vi "Subscriber-3.vi"() -> ()   [LabVIEW 2015]
uses:
  <vilib>/Distrio/LabbitMQ/Channel/exchange_type_enum.ctl
  <vilib>/Distrio/LabbitMQ/Connection/Connection.lvclass
  <vilib>/Distrio/LabbitMQ/Connection/connection_parameters_cluster.ctl
  <vilib>/Distrio/LabbitMQ/Queue/Queue.lvclass
  <vilib>/Distrio/LabbitMQ/Channel/Channel.lvclass
panel:
  in  "buttonStop":bool
  out "Received Message":string
  in  "Subscribe":bool
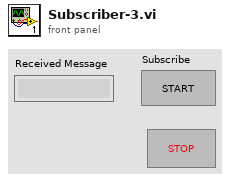
[diagram p1: front panel]
types:
  T1 = typedef "Connection.lvclass/connection_parameters_cluster.ctl" = cluster{"host name":string, "port":i32, "user name":string, "password":string, "virtual host":string}
  T2 = typedef "Channel.lvclass/exchange_type_enum.ctl" = enum16{"direct", "topic", "fanout", "headers"}
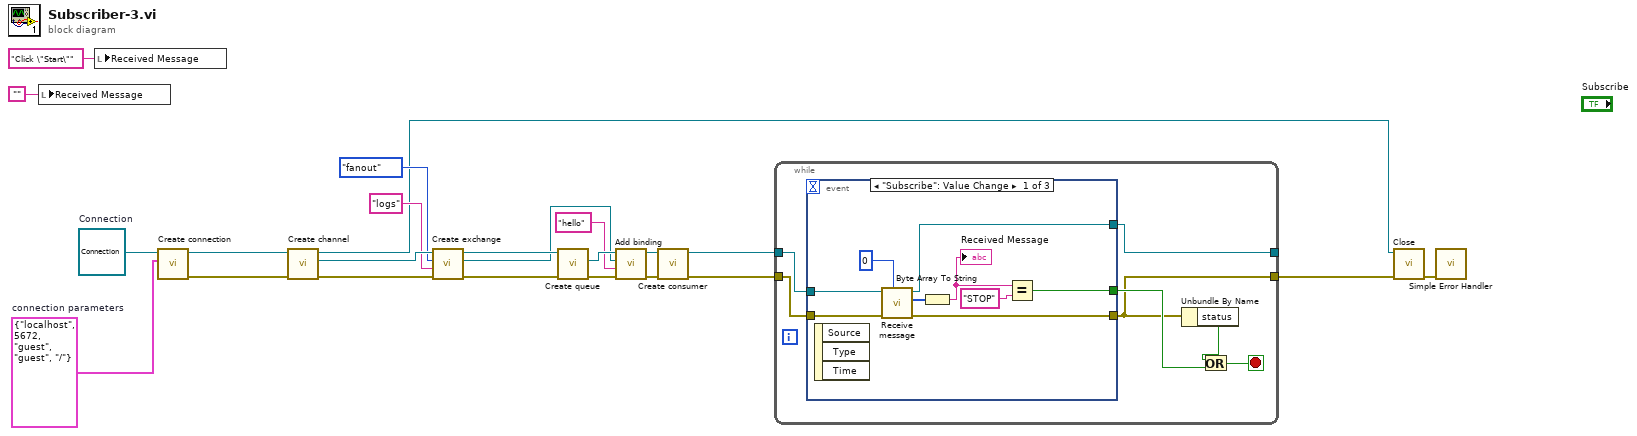
[diagram p0: block diagram]
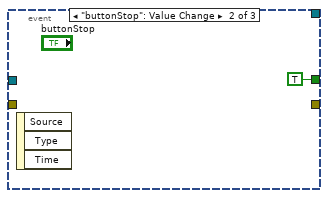
[diagram p2: hidden frame]
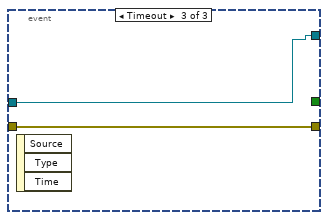
[diagram p3: hidden frame]
diagram:
  w8 = T1 {"host name"="localhost", "port"=5672, "user name"="guest", "password"="guest", "virtual host"="/"}  # connection parameters
  w9 = refnum<class "Connection.lvclass"> refnum  # Connection
  n1 = local write "Received Message"("") -> ()
  n2 = local write "Received Message"("Click \"Start\"") -> ()
  n3 = call <vilib>:"Create connection.vi"("connection parameters"=w8, "Connection in"=w9) -> ("error out"=w22:errorcluster, "Connection out"=w23:refnum<class "Connection.lvclass">)  [unwired: 8 in]
  n4 = call <vilib>:"Create channel.vi"("error in (no error)"=w22, "Connection in"=w23) -> ("error out"=w21:errorcluster, "channel"=w20:refnum<class "Channel.lvclass">, "Connection out"=w7:refnum<class "Connection.lvclass">)  [unwired: 7 in]
  n5 = call <vilib>:"Create exchange.vi"("error in (no error)"=w21, "exchange name"="logs", "exchange type"=exchange_type_enum."fanout" ("binding"), "Channel in"=w20) -> ("error out"=w19:errorcluster, "Exchange.lvclass"=w15:refnum<class "Exchange.lvclass">, "Channel out"=w18:refnum<class "Channel.lvclass">)  [unwired: 5 in]
  n6 = call <vilib>:"Create queue.vi"("error in (no error)"=w19, "Channel in"=w18) -> ("error out"=w17:errorcluster, "Queue.lvclass"=w16:refnum<class "Queue.lvclass">)  [unwired: 7 in, 1 out]
  n7 = call <vilib>:"Add binding.vi"("error in (no error)"=w17, "binding key"="hello" ("routing key"), "Exchange.lvclass"=w15, "Consumer in"=w16) -> ("error out"=w13:errorcluster, "Consumer out"=w12:refnum<class "Queue.lvclass">)  [unwired: 6 in]
  n8 = call <vilib>:"Create consumer.vi"("error in (no error)"=w13, "Queue in"=w12) -> ("error out"=w4:errorcluster, "Queue out"=w5:refnum<class "Queue.lvclass">)  [unwired: 8 in]
  n9 = while {
    tunnel: w5 -> [w30]
    tunnel: w4 -> [w29]
    tunnel: [w25] -> w3
    tunnel: [w28] -> _
    stop <- w26 stop-if-true
    n10 = event shown="[0] \"Subscribe\": Value Change" {
      selector: _ -> [_ _ _]
      dyn-events: _ -> [_ _ _]
      timeout: _ -> [_ _ _]
      tunnel: w30 -> [w38 _ w42]
      tunnel: w29 -> [w37 _ w41]
      tunnel: [w36 _ w42] -> w28
      tunnel: [w34 TRUE _] -> w27
      tunnel: [w33 _ w41] -> w25
      event "Subscribe": Value Change {
        n11 = event-data() -> ()  [unwired: 1 in, 3 out]
        n12 = call <vilib>:"Receive message.vi"("millisecondsTimeout"=0, "error in (no error)"=w37, "Consumer in"=w38) -> ("error out"=w33:errorcluster, "message body"=w39:u8[], "Consumer out"=w36:refnum<class "Queue.lvclass">)  [unwired: 3 in, 3 out]
        n13 = Byte Array To String(unsigned byte array=w39) -> (string=w32:string)
        "Received Message" <- w32
        n14 = Equal?(x=w32, y="STOP") -> (x = y?=w34:bool)
      }
      event "buttonStop": Value Change {
        n15 = event-data() -> ()  [unwired: 1 in, 3 out]
      }
      event Timeout {
        n16 = event-data() -> ()  [unwired: 1 in, 3 out]
      }
    }
    n17 = Unbundle By Name(w25) -> ("status"=w24:bool)
    n18 = Or(x=w24, y=w27) -> (x .or. y?=w26:bool)
  }
  n19 = call <vilib>:"Close.vi"("error in (no error)"=w3, "Connection in"=w7) -> ("error out"=w6:errorcluster)  [unwired: 8 in, 1 out]
  n20 = call <vilib>:"Simple Error Handler.vi"("error in (no error)"=w6) -> ()  [unwired: 4 in, 5 out]
